vi "test_NI 9482.vi"(8 "error in (no error)":errorcluster, 11 "TestCase in":refnum<class "Scan Engine Scripting API Modules.lvclass">) -> (0 "error out":errorcluster, 3 "TestCase out":refnum<class "Scan Engine Scripting API Modules.lvclass">)   [LabVIEW 2019, in "Scan Engine Scripting API Modules.lvclass"]
uses:
  Scan Engine Scripting API Modules.lvclass
  Module Test Classes/NI 9482 Test/NI 9482 Test.lvclass
  <vilib>/addons/_JKI Toolkits/VI Tester/TestCase.llb/TestCase.lvclass
  C:/Program Files (x86)/National Instruments/LabVIEW 2019/vi.lib/addons/_JKI Toolkits/VI Tester/TestCase.llb/TestCase.lvclass
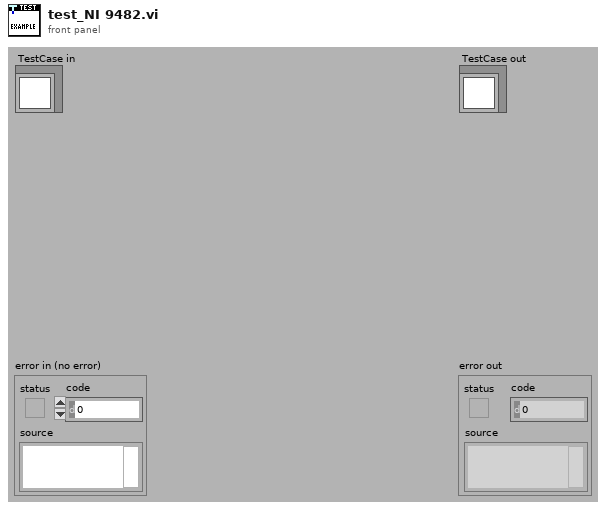
[diagram p1: front panel]
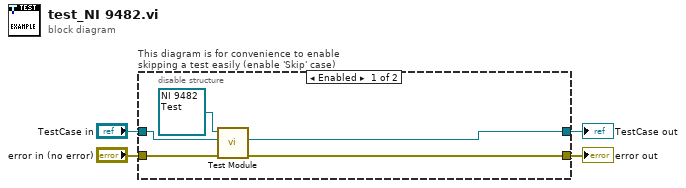
[diagram p0: block diagram]
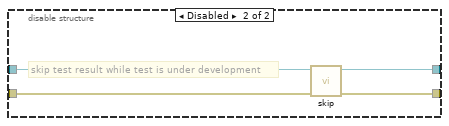
[diagram p2: hidden frame]
diagram:
  n1 = disable-structure "This diagram is for convenience to enable skipping a test easily (enable 'Skip' case)" shown="Enabled" {
    disable-tunnel: "TestCase in" -> [w6 w13]
    disable-tunnel: [w5 w11] -> w1
    disable-tunnel: [w7 w12] -> w3
    disable-tunnel: "error in (no error)" -> [w8 w10]
    frame Enabled {
      n2 = call-dynamic "Test Module.vi"("error in"=w8, "TestCase in"=w6, "module test in"=refnum<class "NI 9482 Test.lvclass"> refnum ("NI 9482 Test.lvclass")) -> ("error out"=w7:errorcluster, "TestCase out"=w5:refnum<class "Scan Engine Scripting API Modules.lvclass">)  [unwired: 6 in, 1 out]
    }
    frame Disabled {
      # "skip test result while test is under development"
      n3 = call <vilib>:"skip.vi"("error in (no error)"=w10, "TestCase in"=w13) -> ("error out"=w12:errorcluster, "TestCase out"=w11:refnum<class "Scan Engine Scripting API Modules.lvclass">)  [unwired: 8 in]
    }
  }
  "error out" <- w3
  "TestCase out" <- w1
